vi "losowe_PH.vi"() -> ()   [LabVIEW 2021]
panel:
  out "Liczby losowe":dbl(graph)
  in  "stop":bool
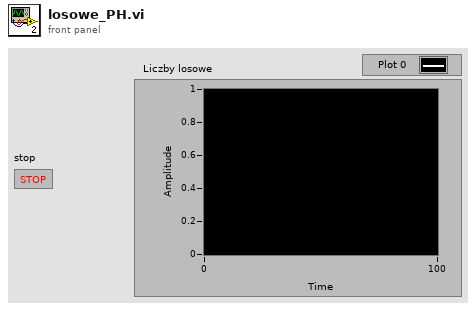
[diagram p1: front panel]
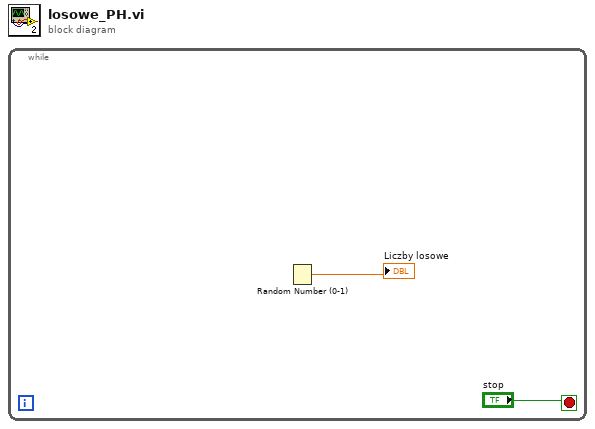
[diagram p0: block diagram]
diagram:
  n1 = while {
    stop <- "stop" stop-if-true
    n2 = Random Number (0-1)() -> (number: 0 to 1=→"Liczby losowe":dbl)
  }
